vi "Get_Centers_Areas_Info_Particles-1.vi"(0 "[IN] Particle Reports (Pixels)":T2(array[cluster]) {"Orientation" format="%.2f"; "Dimensions"."Height" format="%.2f"; "Dimensions"."Width" format="%.2f"; "Center of Mass"."Y" format="%.2f"; "Center of Mass"."X" format="%.2f"; "Bounding Rect"."Bottom" format="%.2f"; "Bounding Rect"."Right" format="%.2f"; "Bounding Rect"."Top" format="%.2f"; "Bounding Rect"."Left" format="%.2f"; "Number of Holes" format="%.2f"; "Area" format="%.2f"}, 1 "error in":errorcluster) -> (2 "[OUT] Array of X,Y":dbl[](array[numeric]), 3 "[OUT] Array of Area":dbl[](array[numeric]), 4 "[OUT] Array of Rectangles":T1(array[cluster]), 5 "error out":errorcluster)   [LabVIEW 2017]
doc: "Get the particle info: (X,Y), area of particle"
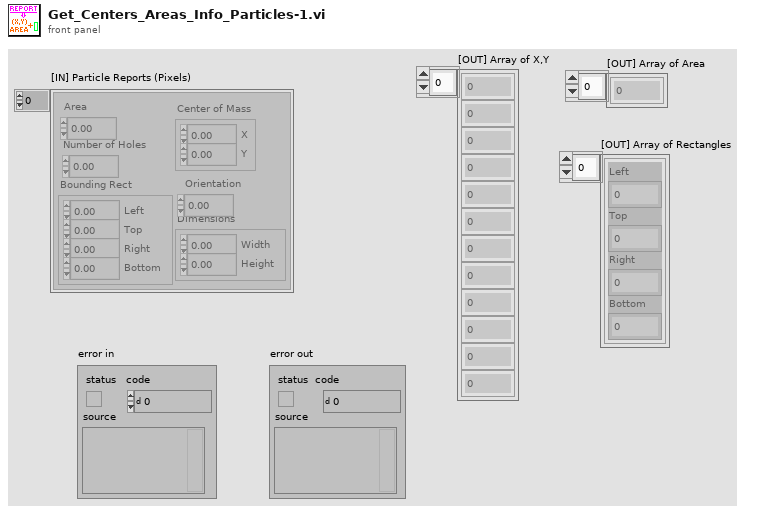
[diagram p1: front panel]
types:
  T1 = cluster{"Left":dbl, "Top":dbl, "Right":dbl, "Bottom":dbl}[]
  T2 = cluster{"Area":dbl, "Number of Holes":dbl, "Bounding Rect":cluster{"Left":dbl, "Top":dbl, "Right":dbl, "Bottom":dbl}, "Center of Mass":cluster{"X":dbl, "Y":dbl}, "Orientation":dbl, "Dimensions":cluster{"Width":dbl, "Height":dbl}}[]
  T3 = cluster{"Left":dbl, "Top":dbl, "Right":dbl, "Bottom":dbl}
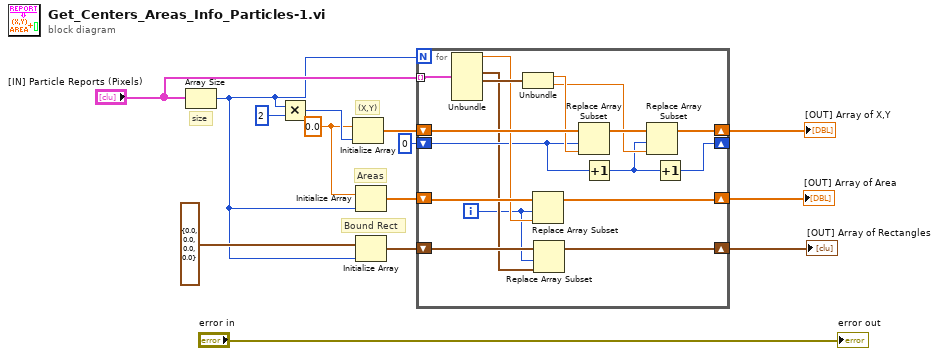
[diagram p0: block diagram]
diagram:
  w7 = 0.0 ("element")
  # "Bound Rect"
  # "size"
  # "Areas"
  # "(X,Y)"
  n1 = Array Size(array="[IN] Particle Reports (Pixels)") -> (size(s)=w3:i32)
  n2 = Multiply(x=w3, y=2) -> (x*y=w13:i32)
  n3 = Initialize Array(w7, w13) -> (w12:dbl[])
  n4 = Initialize Array(w7, w3) -> (w6:dbl[])
  n5 = Initialize Array(T3 {"Left"=0.0, "Top"=0.0, "Right"=0.0, "Bottom"=0.0} ("Bounding Rect"), w3) -> (w2:T1)
  n6 = for {
    N: w3 -> [_]
    tunnel: "[IN] Particle Reports (Pixels)" -> [w31] mode=indexing
    shift-right: [w19] -> _
    shift-left: 0 -> [w21]
    shift-right: [w23] -> w10
    shift-left: w12 -> [w27]
    shift-right: [w28] -> w5
    shift-left: w6 -> [w29]
    shift-right: [w17] -> w1
    shift-left: w2 -> [w18]
    i -> [w15]
    n7 = Unbundle(w31) -> ("Area"=w26:dbl, "Bounding Rect"=w16:T3, "Center of Mass"=w30:cluster{"X":dbl, "Y":dbl})  [unwired: 3 out]
    n8 = Unbundle(w30) -> ("X"=w25:dbl, "Y"=w22:dbl)
    n9 = Replace Array Subset(array=w29, new element=w26, index=w15) -> (w28:dbl[])
    n10 = Replace Array Subset(array=w18, new element=w16, index=w15) -> (w17:T1)
    n11 = Replace Array Subset(array=w27, new element=w25, index=w21) -> (w24:dbl[])
    n12 = Increment(x=w21) -> (x+1=w20:i32)
    n13 = Replace Array Subset(array=w24, new element=w22, index=w20) -> (w23:dbl[])
    n14 = Increment(x=w20) -> (x+1=w19:i32)
  }
  "[OUT] Array of X,Y" <- w10
  "[OUT] Array of Area" <- w5
  "[OUT] Array of Rectangles" <- w1
  "error out" <- "error in"
